vi "repPreparePenaltyEnemyPlayVSS.vi"(8 "error in (no error)":errorcluster, 9 "Game in 2":refnum<class "Game.lvclass">, 10 "RobotPlacement":T1(array[cluster]), 11 "PreparePenaltyEnemyPlayVSS in":refnum<class "PreparePenaltyEnemyPlayVSS.lvclass">) -> (0 "error out":errorcluster, 2 "RobotPlacement 2":T1(array[cluster]), 3 "PreparePenaltyEnemyPlayVSS out":refnum<class "PreparePenaltyEnemyPlayVSS.lvclass">)   [LabVIEW 2023, in "PreparePenaltyEnemyPlayVSS.lvclass"]
uses:
  PreparePenaltyEnemyPlayVSS.lvclass
  Game_class/Game.lvclass
  Game_class/Game.lvclass/Game.ctl
  Game_class/Read FieldRef.vi
  Field_class/Field.lvclass
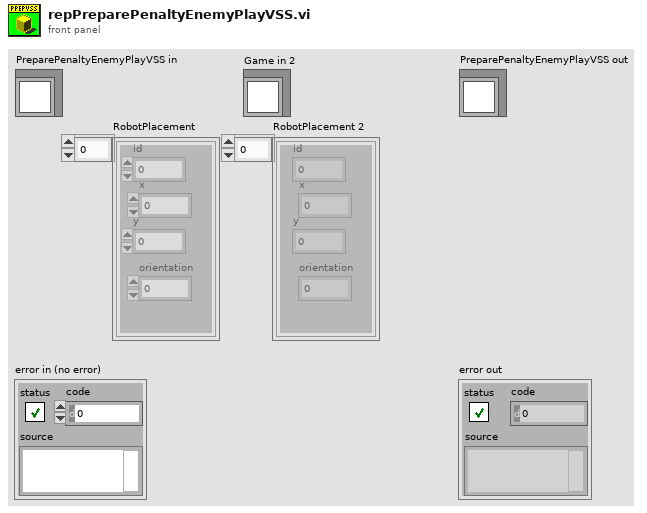
[diagram p1: front panel]
types:
  T1 = cluster{"id":i32, "x":dbl, "y":dbl, "orientation":dbl}[]
  T2 = cluster{"id":i32, "x":dbl, "y":dbl, "orientation":dbl}
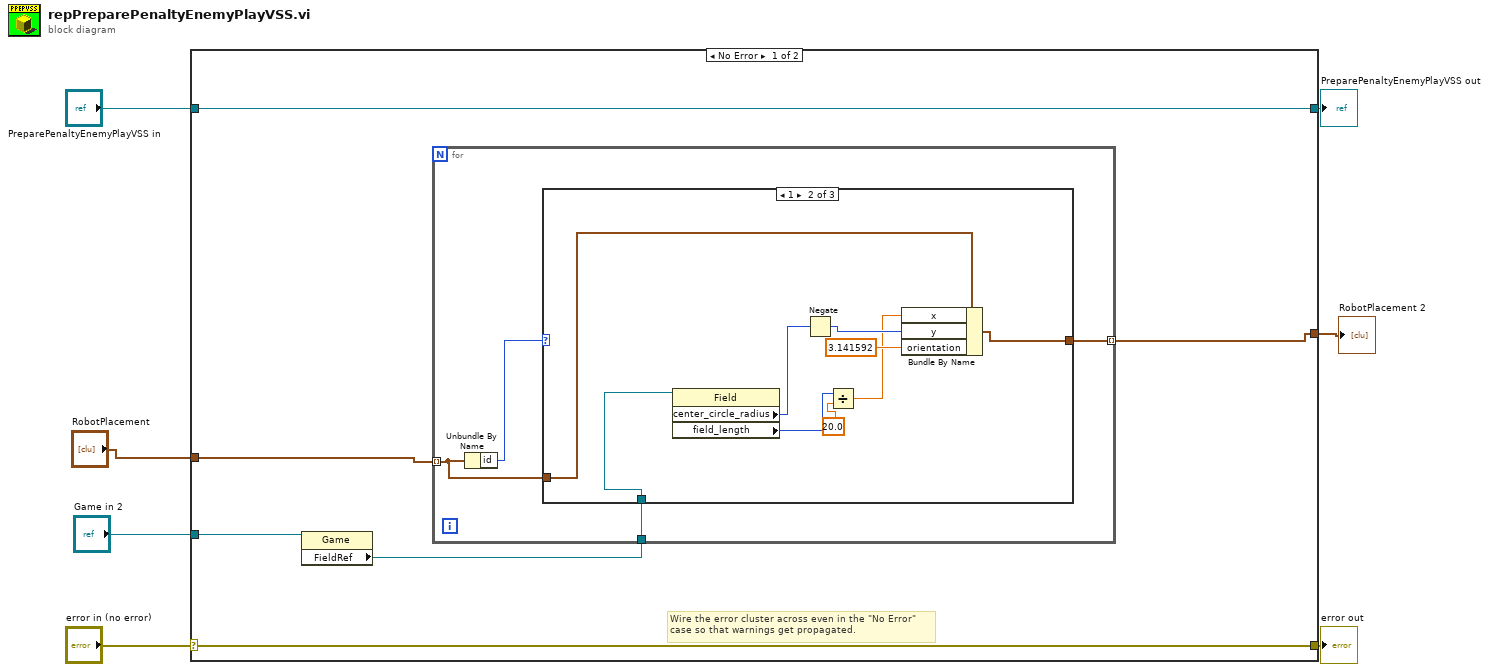
[diagram p0: block diagram]
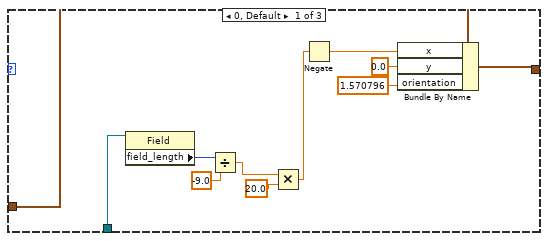
[diagram p2: hidden frame]
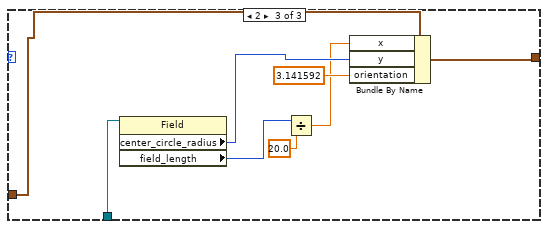
[diagram p3: hidden frame]
diagram:
  n1 = case shown="No Error" "error in (no error)" {
    selector: "error in (no error)" -> [w12 w47]
    tunnel: [w12 w47] -> w6
    tunnel: [w13 w46] -> w4
    tunnel: "PreparePenaltyEnemyPlayVSS in" -> [w13 w46]
    tunnel: [w10 _] -> w3
    tunnel: "RobotPlacement" -> [w9 _]
    tunnel: "Game in 2" -> [w8 _]
    frame No Error {
      # "Wire the error cluster across even in the \"No Error\"\ncase so that warnings get propagated."
      n2 = property class="Game"(reference=w8) -> ("FieldRef"=w11:refnum<class "Field.lvclass">)  [unwired: 1 in, 2 out]
      n3 = for {
        tunnel: w9 -> [w16] mode=indexing
        tunnel: [w15] -> w10 mode=indexing
        tunnel: w11 -> [w14]
        n4 = Unbundle By Name(w16) -> ("id"=w17:i32)
        n5 = case shown="1" w17 {
          tunnel: w16 -> [w28 w37 w44]
          tunnel: [w27 w36 w43] -> w15
          tunnel: w14 -> [w26 w35 w41]
          frame 0, Default {
            n6 = property class="Field"(reference=w26) -> ("field_length"=w25:i32)  [unwired: 1 in, 2 out]
            n7 = Divide(x=w25, y=-9.0) -> (x/y=w20:dbl)
            n8 = Multiply(x=w20, y=20.0) -> (x*y=w19:dbl)
            n9 = Negate(x=w19) -> (-x=w22:dbl)
            n10 = Bundle By Name(cluster=w28, "x"=w22, "y"=0.0, "orientation"=1.570796) -> (w27:T2)
          }
          frame 1 {
            n11 = property class="Field"(reference=w35) -> ("center_circle_radius"=w33:i32, "field_length"=w31:i32)  [unwired: 1 in, 2 out]
            n12 = Negate(x=w33) -> (-x=w32:i32)
            n13 = Divide(x=w31, y=20.0) -> (x/y=w30:dbl)
            n14 = Bundle By Name(cluster=w37, "x"=w30, "y"=w32, "orientation"=3.141592 ("x")) -> (w36:T2)
          }
          frame 2 {
            n15 = property class="Field"(reference=w41) -> ("center_circle_radius"=w42:i32, "field_length"=w40:i32)  [unwired: 1 in, 2 out]
            n16 = Divide(x=w40, y=20.0 ("x")) -> (x/y=w38:dbl)
            n17 = Bundle By Name(cluster=w44, "x"=w38, "y"=w42, "orientation"=3.141592 ("x")) -> (w43:T2)
          }
        }
      }
    }
    frame Error {
    }
  }
  "error out" <- w6
  "PreparePenaltyEnemyPlayVSS out" <- w4
  "RobotPlacement 2" <- w3
